vi "CreateMeanderMask.vi"(7 "Rep. Rate (Hz)":dbl=100.0 min=0.0 max=34.0, 10 "Start Position":dbl[](array[numeric]) min=0.0 max=34.0) -> (0 "BNC_Ctrl":bool, 1 "start/end points":cluster{dbl, dbl}[][](array[cluster]), 2 "Canceled":bool, 5 "ImageParameter":T1)   [LabVIEW 2013]
uses:
  ImagingMS/ImageConvPara.ctl
panel:
  in  "Imaging?":bool
  out "Estimated Time (min)":dbl min=0.0 max=34.0
  in  "Average/pixel":i32=10 min=0 max=34
  in  "Apply":bool
  in  "Cancel":bool
  in  "Run":bool
  out "XY Graph":cluster{dbl, dbl}[](graph)
  out "Y Size (mm)":dbl min=0.0 max=34.0
  out "X Size (mm)":dbl min=0.0 max=34.0
  in  "Y Steps":i32=40 min=0 max=34
  in  "X Size":dbl=2.0 min=0.0 max=34.0
  in  "Y StepWidth":dbl=0.05 min=0.0 max=34.0
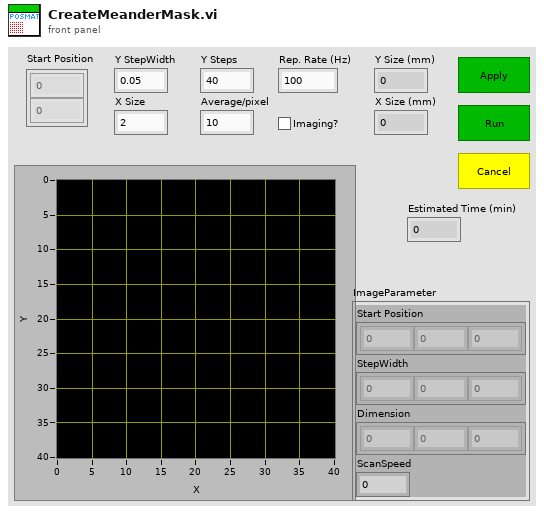
[diagram p1: front panel]
types:
  T1 = typedef "ImageConvPara.ctl" = cluster{"Start Position":dbl[], "StepWidth":dbl[], "Dimension":i32[], "ScanSpeed":dbl}
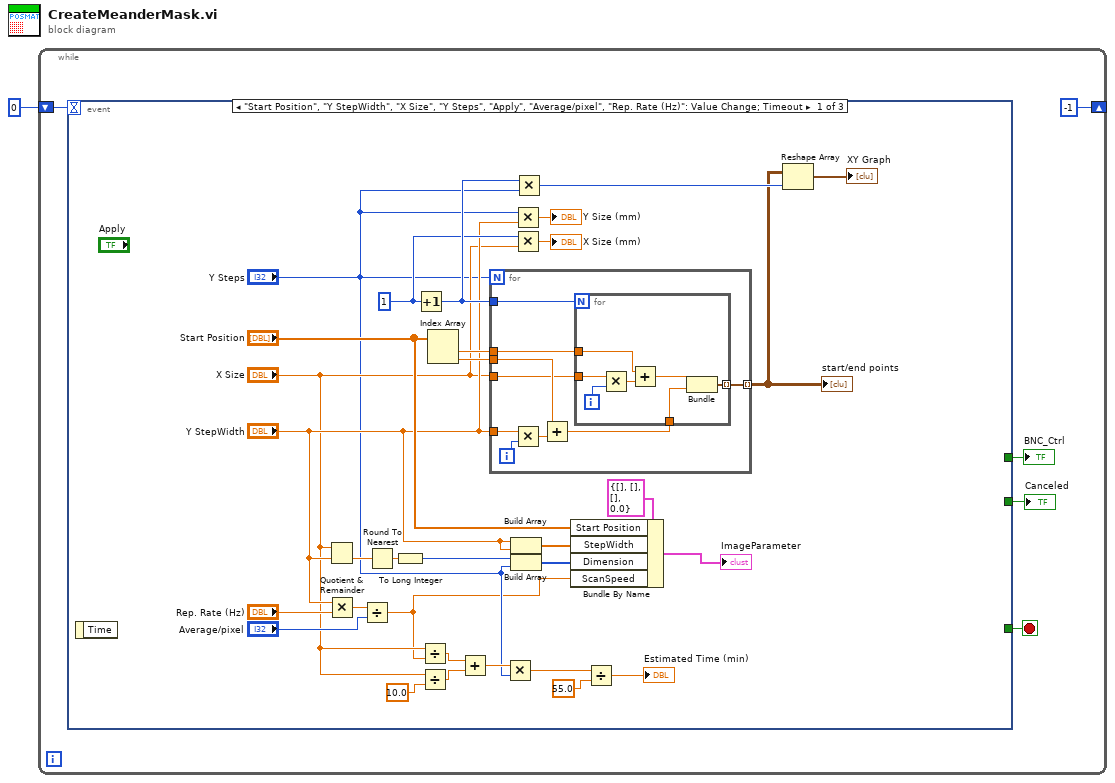
[diagram p0: block diagram]
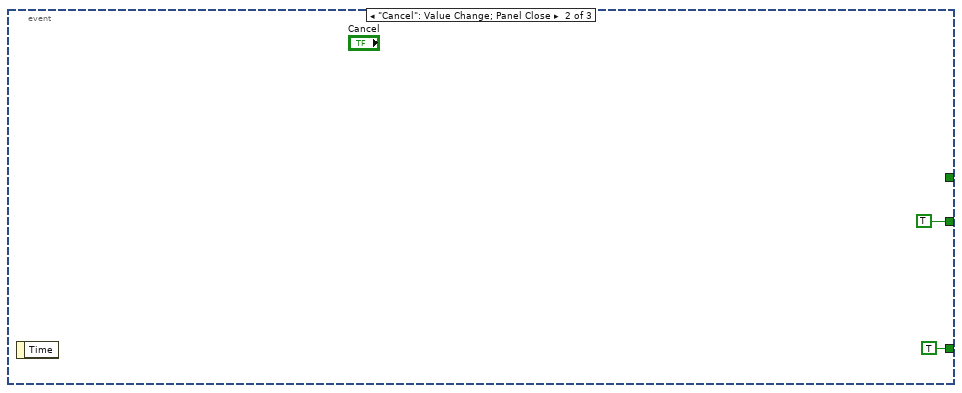
[diagram p2: hidden frame]
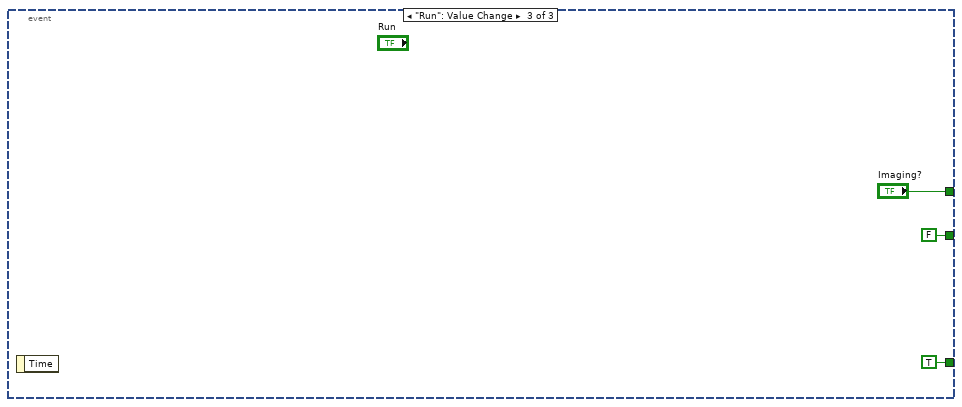
[diagram p3: hidden frame]
diagram:
  n1 = while {
    shift-right: [-1] -> _
    shift-left: 0 -> [w2]
    stop <- w6 stop-if-true
    n2 = event shown="[0] \"Start Position\", \"Y StepWidth\", \"X Size\", \"Y Steps\", \"Apply\", \"Average/pixel\", \"Rep. Rate (Hz)\": Value Change;  Timeout" {
      selector: _ -> [_ _ _]
      dyn-events: _ -> [_ _ _]
      timeout: w2 -> [_ _ _]
      tunnel: [_ TRUE TRUE] -> w6
      tunnel: [_ TRUE ("Canceled") FALSE ("Canceled")] -> w5
      tunnel: [_ _ "Imaging?"] -> w4
      event "Start Position", "Y StepWidth", "X Size", "Y Steps", "Apply", "Average/pixel", "Rep. Rate (Hz)": Value Change; Timeout {
        w31 = 1
        n3 = event-data() -> ()  [unwired: 1 in, 1 out]
        n4 = Quotient & Remainder(x="X Size", y="Y StepWidth") -> (floor(x/y)=w23:dbl)  [unwired: 1 out]
        n5 = Multiply(x="Y StepWidth", y="Rep. Rate (Hz)") -> (x*y=w22:dbl)
        n6 = Divide(x=w22, y="Average/pixel") -> (x/y=w9:dbl)
        n7 = Round To Nearest(number=w23) -> (nearest integer value=w7:dbl)
        n8 = To Long Integer(number=w7) -> (32bit integer=w8:i32)
        n9 = Increment(x=w31) -> (x+1=w32:i32)
        n10 = Divide(x="X Size", y=w9) -> (x/y=w17:dbl)
        n11 = Divide(x="X Size", y=10.0) -> (x/y=w16:dbl)
        n12 = Index Array(array="Start Position") -> (element #1=w37:dbl, element #2=w36:dbl)  [unwired: 2 in]
        n13 = Add(x=w17, y=w16) -> (x+y=w15:dbl)
        n14 = for {
          N: "Y Steps" -> [_]
          tunnel: w37 -> [w38]
          tunnel: w36 -> [w40]
          tunnel: "Y StepWidth" -> [w45]
          tunnel: "X Size" -> [w39]
          tunnel: w32 -> [w42]
          tunnel: [w41] -> w29 mode=indexing
          i -> [w46]
          n15 = Multiply(x=w45, y=w46) -> (x*y=w44:dbl)
          n16 = Add(x=w40, y=w44) -> (x+y=w43:dbl)
          n17 = for {
            N: w42 -> [_]
            tunnel: w39 -> [w51]
            tunnel: w38 -> [w50]
            tunnel: w43 -> [w48]
            tunnel: [w49] -> w41 mode=indexing
            i -> [w52]
            n18 = Multiply(x=w51, y=w52) -> (x*y=w53:dbl)
            n19 = Add(x=w50, y=w53) -> (x+y=w47:dbl)
            n20 = Bundle(w47, w48) -> (w49:cluster{dbl, dbl})  [unwired: 1 in]
          }
        }
        "start/end points" <- w29
        n21 = Multiply(x=w15, y="Y Steps") -> (x*y=w14:dbl)
        n22 = Build Array("Y StepWidth", "Y StepWidth") -> (w26:dbl[])
        n23 = Build Array(w8, "Y Steps") -> (w25:i32[])
        n24 = Multiply(x="Y Steps", y="Y StepWidth") -> (x*y=→"Y Size (mm)":dbl)
        n25 = Multiply(x=w31, y="X Size") -> (x*y=→"X Size (mm)":dbl)
        n26 = Multiply(x=w32, y="Y Steps") -> (x*y=w33:i32)
        n27 = Bundle By Name(cluster=T1 {"Start Position"=[], "StepWidth"=[], "Dimension"=[], "ScanSpeed"=0.0} ("ImageParameter"), "Start Position"="Start Position", "StepWidth"=w26, "Dimension"=w25, "ScanSpeed"=w9) -> (→"ImageParameter":T1)
        n28 = Divide(x=w14, y=55.0) -> (x/y=→"Estimated Time (min)":dbl)
        n29 = Reshape Array(w29, w33) -> (→"XY Graph":cluster{dbl, dbl}[])
      }
      event "Cancel": Value Change; Panel Close {
        n30 = event-data() -> ()  [unwired: 1 in, 1 out]
      }
      event "Run": Value Change {
        n31 = event-data() -> ()  [unwired: 1 in, 1 out]
      }
    }
    "Canceled" <- w5
    "BNC_Ctrl" <- w4
  }
